vi "Log (WARNING).vi"(8 "Error in (no error)":errorcluster, 10 "Message":string, 11 "Log in":refnum<class "Log.lvclass">) -> (0 "Error out":errorcluster, 3 "Log out":refnum<class "Log.lvclass">)   [LabVIEW 2011, in "Log.lvclass"]
uses:
  Log.lvclass
  LogCluster.ctl
  PrioritiesRing.ctl
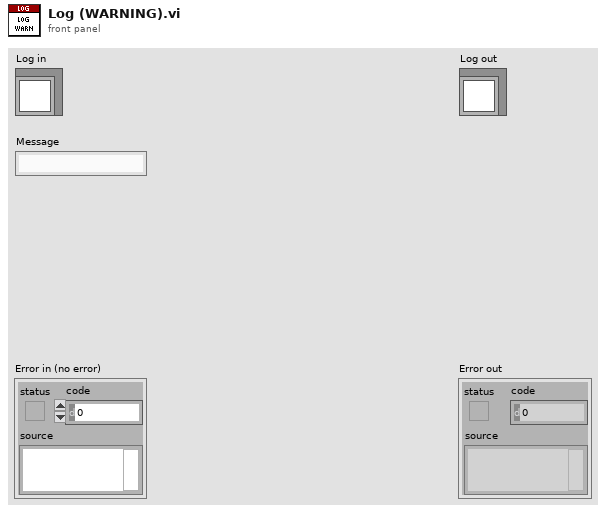
[diagram p1: front panel]
types:
  T1 = typedef "Log.lvclass/PrioritiesRing.ctl" = u32
  T2 = typedef "Log.lvclass/LogCluster.ctl" = cluster{"Timestamp":string, "Message":string, "Priority":T1, "PriorityName":string}
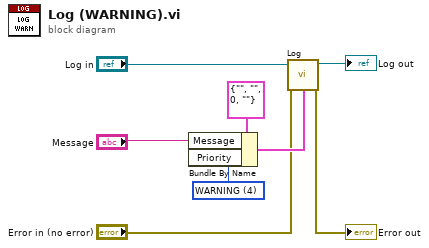
[diagram p0: block diagram]
diagram:
  w6 = T1 4 items=["EMERGENCY", "ALERT", "CRITICAL", "ERROR", "WARNING", "NOTICE", "INFO", "DEBUG"] ("Ring")
  n1 = Bundle By Name(cluster=T2 {"Timestamp"="", "Message"="", "Priority"=0, "PriorityName"=""} ("Log"), "Message"="Message", "Priority"=w6) -> (w5:T2)
  n2 = call "Log.vi"("Error in (no error)"="Error in (no error)", 10:"Log in"=w5, 11:"Log in"="Log in") -> ("Error out"=→"Error out":errorcluster, "Log out"=→"Log out":refnum<class "Log.lvclass">)  [unwired: 7 in]
